vi "Get Device Type.vi"(8 "Error In":errorcluster, 11 "Install LV Data":T1) -> (0 "Error Out":errorcluster, 2 "Device Type":string, 3 "Install LV Data":T1)   [LabVIEW 2014, in "LMH-LINX.lvlib"]
uses:
  <vilib>/MakerHub/LINX/LMH-LINX.lvlib
  <vilib>/MakerHub/LINX/Private/Utilties/Target Management/Install LV Data.ctl
  C:/Program Files (x86)/National Instruments/LabVIEW 2014/vi.lib/MakerHub/LINX/Resources/Renci.SshNet.dll
  Resources/Renci.SshNet.dll
  <vilib>/MakerHub/LINX/Private/Utilties/Target Management/Target Info.ctl
  <vilib>/MakerHub/LINX/Private/Utilties/Target Management/NIC Info.ctl
  <vilib>/MakerHub/LINX/Private/Utilties/Target Management/NIC Mode.ctl
  <vilib>/regexp/Match Regular Expression.xnode
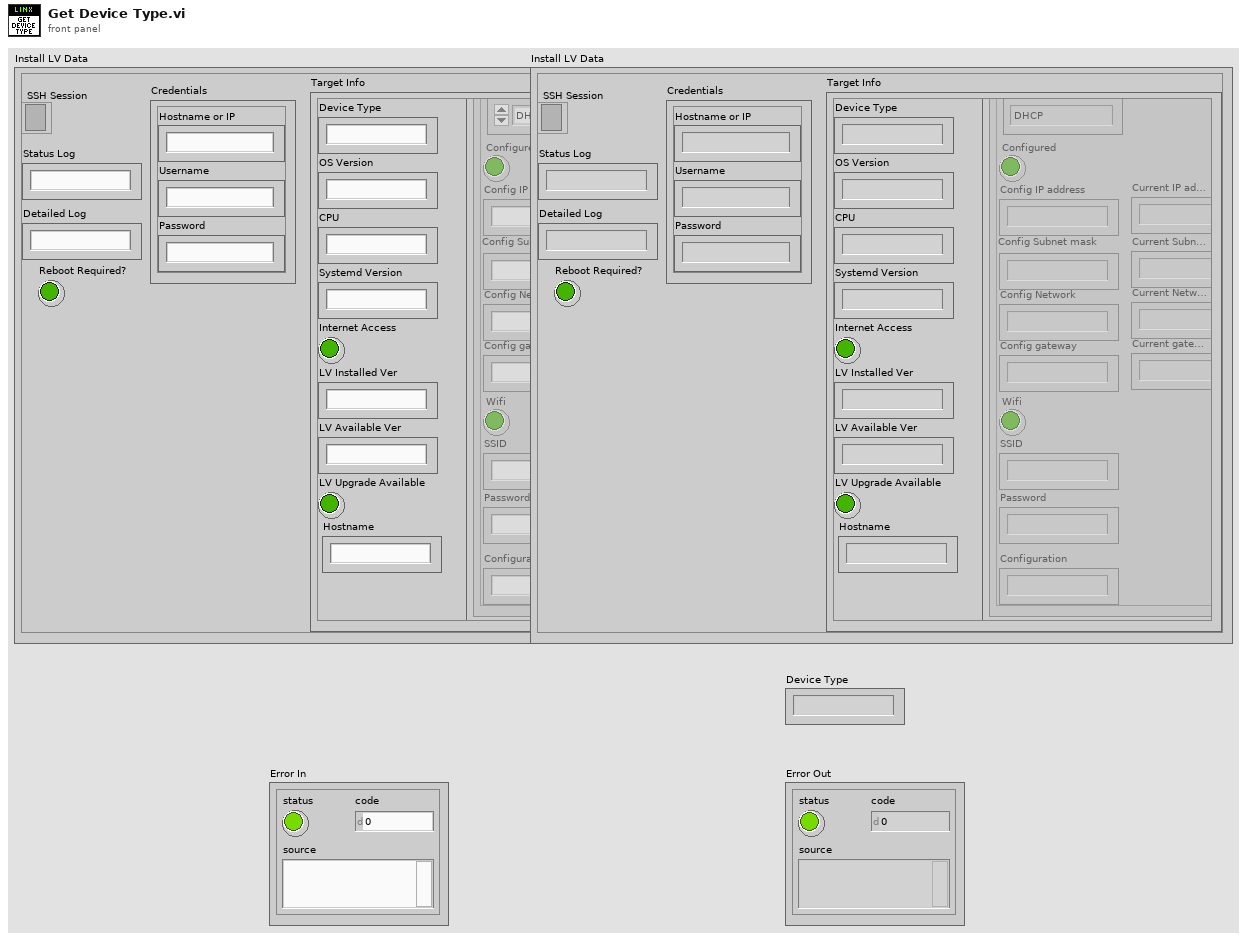
[diagram p1: front panel]
types:
  T1 = typedef "LMH-LINX.lvlib/Install LV Data.ctl" = cluster{"SSH Session":refnum<k24>, "Status Log":string, "Detailed Log":string, "Credentials":cluster{"Hostname or IP":string, "Username":string, "Password":string}, "Target Info":T2, "Reboot Required?":bool}
  T2 = typedef "LMH-LINX.lvlib/Target Info.ctl" = cluster{"OS Version":string, "CPU":string, "Systemd Version":string, "Internet Access":bool, "Device Type":string, "LV Installed Ver":string, "LV Available Ver":string, "LV Upgrade Available":bool, "Hostname":string, "NIC Info":T3[]}
  T3 = typedef "LMH-LINX.lvlib/NIC Info.ctl" = cluster{"Name":string, "NIC Mode":T4, "Configured":bool, "Config IP address":string, "Config Subnet mask":string, "Config Network":string, "Config gateway":string, "Wifi":bool, "SSID":string, "Password":string, "Configuration":string, "Current IP address":string, "Current Subnet mask":string, "Current gateway":string, "Current Network":string}
  T4 = typedef "LMH-LINX.lvlib/NIC Mode.ctl" = enum16{"DHCP", "Static", "Loopback"}
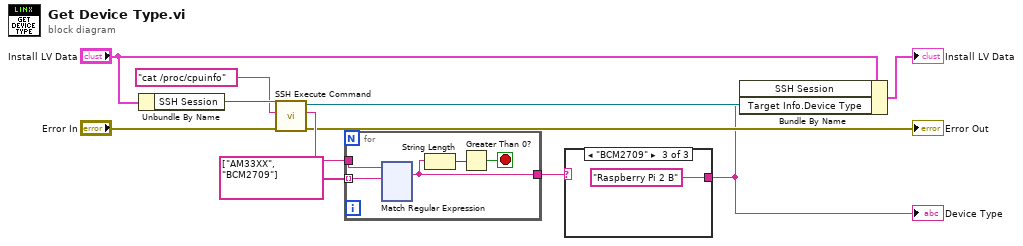
[diagram p0: block diagram]
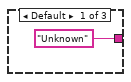
[diagram p2: hidden frame]
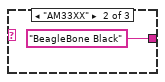
[diagram p3: hidden frame]
diagram:
  n1 = Unbundle By Name("Install LV Data") -> ("SSH Session"=w11:refnum<k24>)
  n2 = call <vilib>:"SSH Execute Command.vi"("Error In"="Error In", "Command"="cat /proc/cpuinfo", "SSH Session"=w11) -> ("Error Out"=→"Error Out":errorcluster, "Std Out"=w7:string, "SSH Session"=w4:refnum<k24>)  [unwired: 6 in]
  n3 = for {
    tunnel: w7 -> [w16]
    tunnel: string[] ["AM33XX", "BCM2709"] -> [w14] mode=indexing
    tunnel: [w12] -> w9
    stop <- w13 stop-if-true
    n4 = xnode "Match Regular Expression"("input string"=w16, "regular expression"=w14) -> ("whole match"=w12:string)  [unwired: 4 in, 4 out]
    n5 = String Length(string=w12) -> (length=w15:i32)
    n6 = Greater Than 0?(x=w15) -> (x > 0?=w13:bool)
  }
  n7 = case shown="\"BCM2709\"" w9 {
    tunnel: ["Unknown" ("regular expression") "BeagleBone Black" ("regular expression") "Raspberry Pi 2 B" ("regular expression")] -> w3
    frame Default {
    }
    frame "AM33XX" {
    }
    frame "BCM2709" {
    }
  }
  "Device Type" <- w3
  n8 = Bundle By Name(cluster="Install LV Data", "SSH Session"=w4, "Target Info.Device Type"=w3) -> (→"Install LV Data":T1)
